vi "生产统计数据Main.vi"(6 "错误in":errorcluster caption="错误常量", 7 "图像处理结果(in)":bool, 8 "产品型号":string="高速插头Gap", 9 "生产统计数据操作":T2) -> (0 "错误out":errorcluster caption="错误常量", 1 "3生产统计-复锁拍螺帽":T1 {"良率" format="%#.2g"}, 2 "2生产统计-取料拍螺帽":T1 {"良率" format="%#.2g"}, 3 "1生产统计-拍PCB孔":T1 {"良率" format="%#.2g"})   [LabVIEW 2014]
uses:
  Controls/ProductNum.ctl
panel:
  # "%"
  # "%"
  # "%"
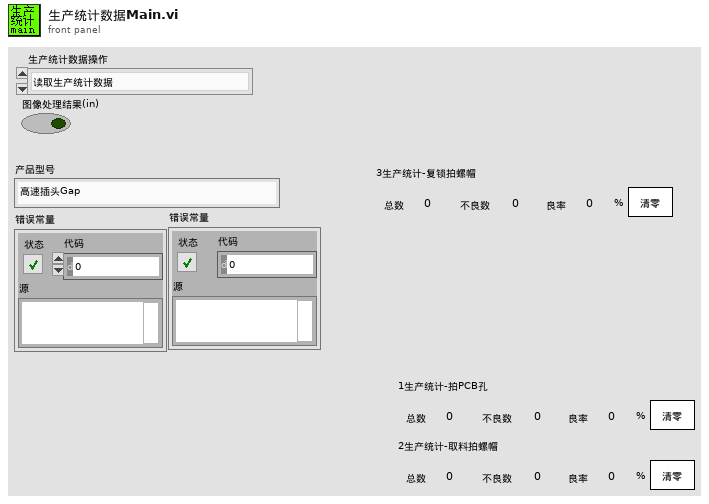
[diagram p1: front panel]
types:
  T1 = typedef "ProductNum.ctl" = cluster{"总数":u64, "不良数":u64, "良率":dbl, "清零":bool}
  T2 = typedef "控件-生产统计数据动作.ctl" = enum16{"读取生产统计数据", "更新并保存拍PCB孔生产数据", "更新并保存取料拍螺帽生产数据", "更新并保存复锁拍螺帽生产数据", "清零拍PCB孔生产数据", "清零取料拍螺帽生产数据", "清零复锁拍螺帽生产数据"}
  T3 = typedef "控件-拍照内容.ctl" = enum16{"拍PCB孔", "取料拍螺帽", "复锁拍螺帽"}
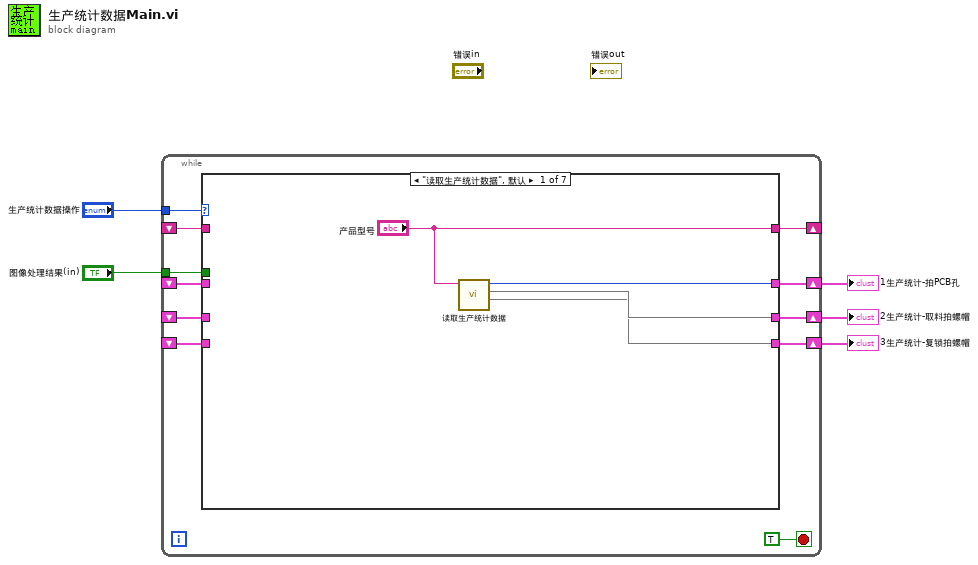
[diagram p0: block diagram]
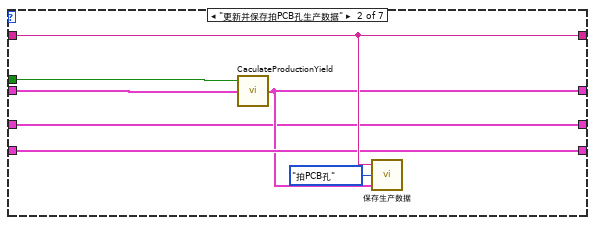
[diagram p2: hidden frame]
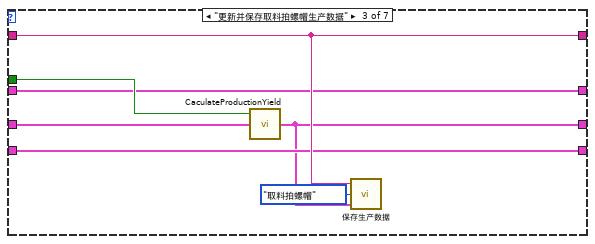
[diagram p3: hidden frame]
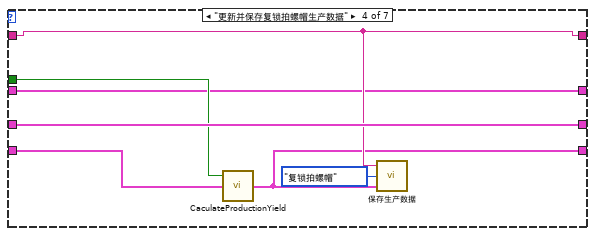
[diagram p4: hidden frame]
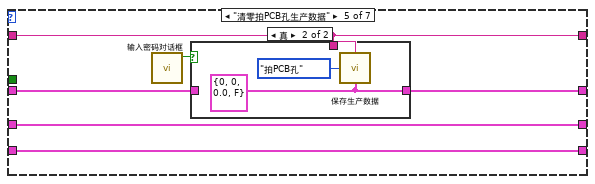
[diagram p5: hidden frame]
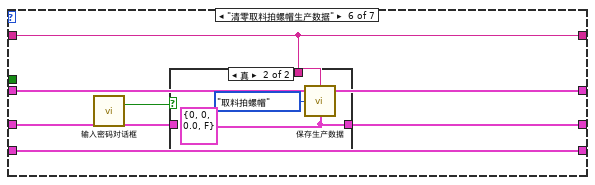
[diagram p7: hidden frame]
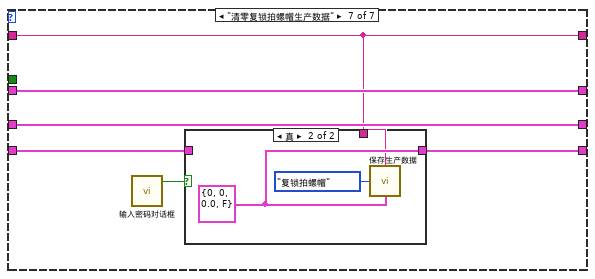
[diagram p9: hidden frame]
diagram:
  n1 = while {
    tunnel: "生产统计数据操作" -> [w15]
    shift-right: [w14] -> _
    shift-left: _ -> [w8]
    shift-right: [w13] -> w4
    shift-left: _ -> [w11]
    shift-right: [w12] -> w3
    shift-left: _ -> [w9]
    tunnel: "图像处理结果(in)" -> [w10]
    shift-right: [w7] -> w1
    shift-left: _ -> [w6]
    stop <- TRUE stop-if-true
    n2 = case shown="\"读取生产统计数据\", 默认" w15 {
      tunnel: ["产品型号" w26 w33 w39 w47 w57 w64] -> w14
      tunnel: [w19 w22 w29 w37 w45 w54 w67] -> w13
      tunnel: [w18 w21 w28 w40 w44 w55 w66] -> w12
      tunnel: w11 -> [_ w23 w29 w37 w42 w54 w67]
      tunnel: w10 -> [_ w27 w34 w38 _ _ _]
      tunnel: w9 -> [_ w21 w30 w40 w44 w52 w66]
      tunnel: w8 -> [_ w26 w33 w39 w47 w57 w64]
      tunnel: [w17 w24 w31 w35 w46 w56 w65] -> w7
      tunnel: w6 -> [_ w24 w31 w36 w46 w56 w62]
      frame "读取生产统计数据", Default {
        n3 = call "读取生产统计数据.vi"("产品码"="产品型号") -> (1:w17, 2:w18, "线号"=w19:i32)  [unwired: 6 in]
      }
      frame "更新并保存拍PCB孔生产数据" {
        n4 = call "CaculateProductionYield.vi"("生产统计"=w23, "Result(in)"=w27) -> ("良率统计out"=w22:T1)  [unwired: 1 in]
        n5 = call "保存生产数据.vi"("error out"=w22, 1:控件-拍照内容."拍PCB孔" ("选择拍照内容"), "输入簇"=w26) -> ()
      }
      frame "更新并保存取料拍螺帽生产数据" {
        n6 = call "CaculateProductionYield.vi"("生产统计"=w30, "Result(in)"=w34) -> ("良率统计out"=w28:T1)  [unwired: 1 in]
        n7 = call "保存生产数据.vi"("error out"=w28, 1:控件-拍照内容."取料拍螺帽" ("选择拍照内容"), "输入簇"=w33) -> ()
      }
      frame "更新并保存复锁拍螺帽生产数据" {
        n8 = call "CaculateProductionYield.vi"("生产统计"=w36, "Result(in)"=w38) -> ("良率统计out"=w35:T1)  [unwired: 1 in]
        n9 = call "保存生产数据.vi"("error out"=w35, 1:控件-拍照内容."复锁拍螺帽" ("选择拍照内容"), "输入簇"=w39) -> ()
      }
      frame "清零拍PCB孔生产数据" {
        n10 = call "输入密码对话框.vi"() -> ("密码正确"=w43:bool)  [unwired: 11 in]
        n11 = case shown="真" w43 {
          tunnel: w47 -> [_ w50]
          tunnel: [w48 w49] -> w45
          tunnel: w42 -> [w48 _]
          frame False {
          }
          frame True {
            w49 = T1 {"总数"=0, "不良数"=0, "良率"=0.0, "清零"=FALSE} ("良率统计")
            n12 = call "保存生产数据.vi"("error out"=w49, 1:控件-拍照内容."拍PCB孔" ("选择拍照内容"), "输入簇"=w50) -> ()
          }
        }
      }
      frame "清零取料拍螺帽生产数据" {
        n13 = call "输入密码对话框.vi"() -> ("密码正确"=w53:bool)  [unwired: 11 in]
        n14 = case shown="真" w53 {
          tunnel: w57 -> [_ w60]
          tunnel: [w58 w59] -> w55
          tunnel: w52 -> [w58 _]
          frame False {
          }
          frame True {
            w59 = T1 {"总数"=0, "不良数"=0, "良率"=0.0, "清零"=FALSE} ("良率统计")
            n15 = call "保存生产数据.vi"("error out"=w59, 1:控件-拍照内容."取料拍螺帽" ("选择拍照内容"), "输入簇"=w60) -> ()
          }
        }
      }
      frame "清零复锁拍螺帽生产数据" {
        n16 = call "输入密码对话框.vi"() -> ("密码正确"=w63:bool)  [unwired: 11 in]
        n17 = case shown="真" w63 {
          tunnel: [w68 w70] -> w65
          tunnel: w64 -> [_ w69]
          tunnel: w62 -> [w68 _]
          frame False {
          }
          frame True {
            w70 = T1 {"总数"=0, "不良数"=0, "良率"=0.0, "清零"=FALSE} ("良率统计")
            n18 = call "保存生产数据.vi"("error out"=w70, 1:控件-拍照内容."复锁拍螺帽" ("选择拍照内容"), "输入簇"=w69) -> ()
          }
        }
      }
    }
  }
  "1生产统计-拍PCB孔" <- w4
  "2生产统计-取料拍螺帽" <- w3
  "3生产统计-复锁拍螺帽" <- w1
